vi "Send Message to Websockets.vi"(8 "Error In":errorcluster, 10 "Data":string, 11 "Command":string) -> (0 "error out":errorcluster)   [LabVIEW 2014]
uses:
  Controls/Websocket Data.ctl
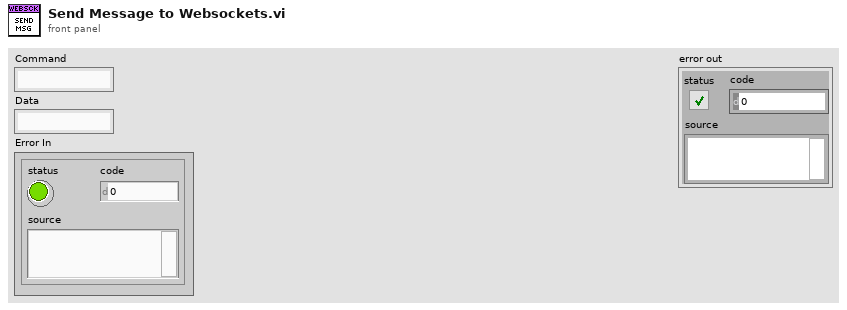
[diagram p1: front panel]
types:
  T1 = typedef "Websocket Data.ctl" = cluster{"Command":string, "Data":string}
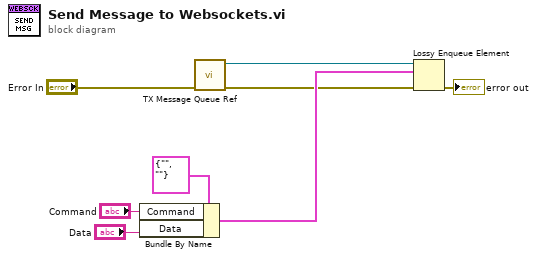
[diagram p0: block diagram]
diagram:
  n1 = Bundle By Name(cluster=T1 {"Command"="", "Data"=""} ("Websocket Data"), "Command"="Command", "Data"="Data") -> (w4:T1)
  n2 = call "TX Message Queue Ref.vi"("Error In"="Error In") -> ("error out"=w2:errorcluster, "tx queue ref"=w8:refnum<queue>)  [unwired: 9 in]
  n3 = Lossy Enqueue Element(queue=w8, element=w4, error in (no error)=w2) -> (error out=→"error out":errorcluster)  [unwired: 3 out]
